vi "first_row_labels.vi"() -> (3 "Array":string[](array[string]))   [LabVIEW 2014]
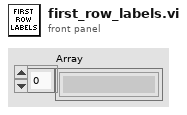
[diagram p1: front panel]
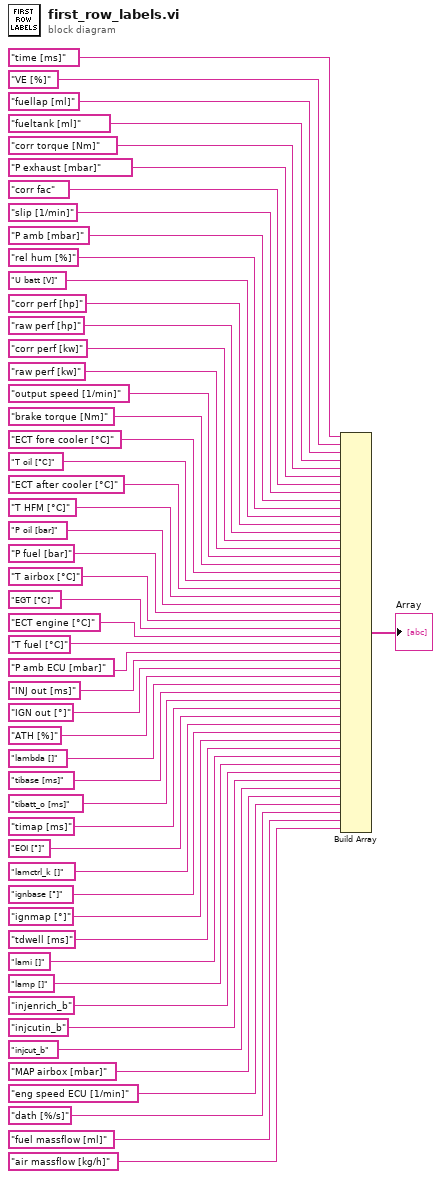
[diagram p0: block diagram]
diagram:
  n1 = Build Array("time [ms]" ("element"), "VE [%]" ("element"), "fuellap [ml]" ("element"), "fueltank [ml]" ("element"), "corr torque [Nm]" ("element"), "P exhaust [mbar]" ("element"), "corr fac", "slip [1/min]", "P amb [mbar]", "rel hum [%]", "U batt [V]", "corr perf [hp]", "raw perf [hp]", "corr perf [kw]", "raw perf [kw]", "output speed [1/min]", "brake torque [Nm]", "ECT fore cooler [°C]", "T oil [°C]", "ECT after cooler [°C]", "T HFM [°C]", "P oil [bar]", "P fuel [bar]", "T airbox [°C]", "EGT [°C]", "ECT engine [°C]", "T fuel [°C]", "P amb ECU [mbar]", "INJ out [ms]", "IGN out [°]", "ATH [%]", "lambda []", "tibase [ms]", "tibatt_o [ms]", "timap [ms]", "EOI [°]", "lamctrl_k []", "ignbase [°]", "ignmap [°]", "tdwell [ms]", "lami []", "lamp []", "injenrich_b", "injcutin_b", "injcut_b", "MAP airbox [mbar]", "eng speed ECU [1/min]", "dath [%/s]", "fuel massflow [ml]", "air massflow [kg/h]") -> (→"Array":string[])
